vi "Write Log Message Enqueuer.vi"(8 "error in (no error)":errorcluster caption="错误输入（无错误）", 10 "操作者框架:消息待入队列":refnum<class "Message Enqueuer.lvclass">, 11 "ErrorHanlder输入":refnum<class "ErrorHanlder.lvclass">) -> (0 "error out":errorcluster caption="错误输出", 3 "ErrorHanlder输出":refnum<class "ErrorHanlder.lvclass">)   [LabVIEW 2018, in "ErrorHanlder.lvlib" / "ErrorHanlder.lvclass"]
uses:
  ErrorHanlder.lvclass
  <vilib>/ActorFramework/Message Enqueuer/Message Enqueuer.lvclass
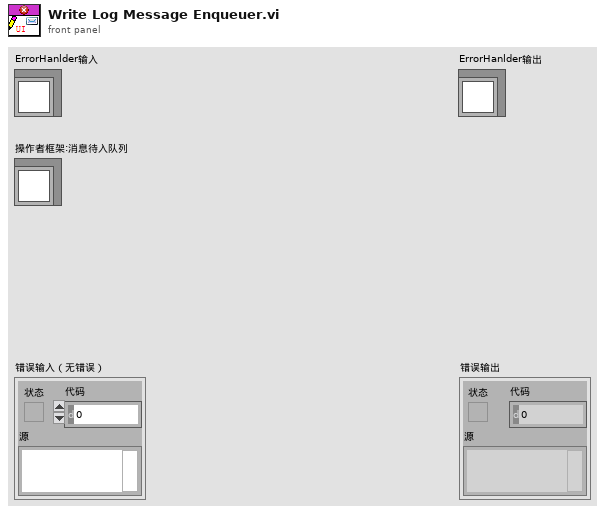
[diagram p1: front panel]
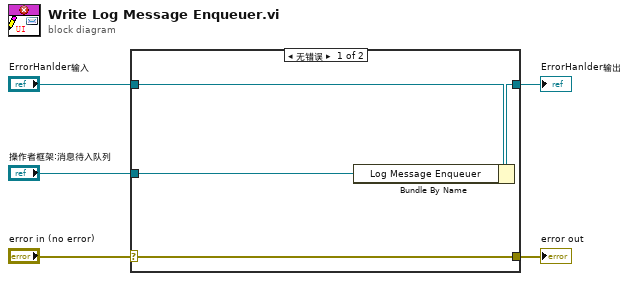
[diagram p0: block diagram]
diagram:
  n1 = case shown="无错误" "error in (no error)" {
    selector: "error in (no error)" -> [w9 w10]
    tunnel: [w9 w10] -> w4
    tunnel: [w7 w11] -> w2
    tunnel: "ErrorHanlder输入" -> [w8 w11]
    tunnel: "操作者框架:消息待入队列" -> [w6 _]
    frame No Error {
      n2 = Bundle By Name(cluster=w8, "Log Message Enqueuer"=w6) -> (w7:refnum<class "ErrorHanlder.lvclass">)
    }
    frame Error {
    }
  }
  "error out" <- w4
  "ErrorHanlder输出" <- w2
